vi "runBraking.vi"(6 "Fault?":bool, 7 "x acceleration":dbl, 8 "error in (no error)":errorcluster, 9 "Actuators in":T1, 10 "State in":T2, 11 "SystemsCheck in":refnum<class "SystemsCheck.lvclass">) -> (0 "error out":errorcluster, 1 "Actuators out":T1, 2 "State out":T2, 3 "SystemsCheck out":refnum<class "SystemsCheck.lvclass">)   [LabVIEW 2017, in "ControlLibrary.lvlib" / "SystemsCheck.lvclass"]
uses:
  SystemsCheck.lvclass
  TypeDef_ControlState.ctl
  TypeDef_DigitalOuts.ctl
  RunTypeClass/RunType.lvclass
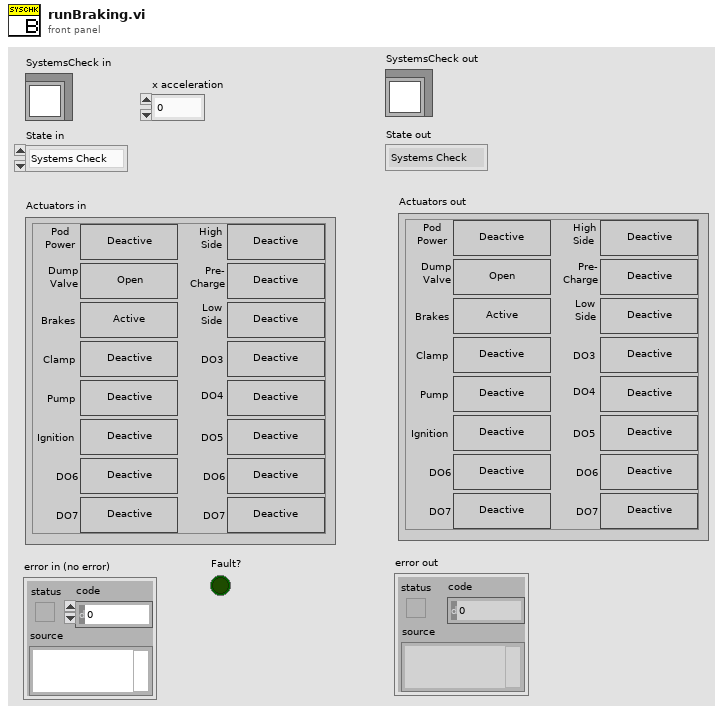
[diagram p1: front panel]
types:
  T1 = typedef "TypeDef_DigitalOuts.ctl" = cluster{"Pod Power":bool, "Dump Valve":bool, "Brakes":bool, "Clamp":bool, "Pump":bool, "Ignition":bool, "DO6":bool, "DO7":bool, "HighSide":bool, "Precharge":bool, "LowSide":bool, "DO3":bool, "DO4":bool, "DO5":bool, "DO62":bool, "DO72":bool}
  T2 = typedef "TypeDef_ControlState.ctl" = enum16{"Systems Check", "Idle", "Ready", "Pushing", "Coast", "Braking", "Fault", "Shutdown", "Service", "Precharge", "Blank"}
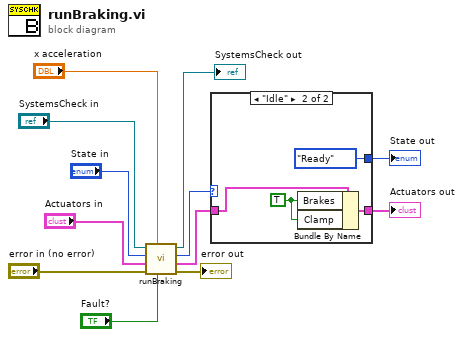
[diagram p0: block diagram]
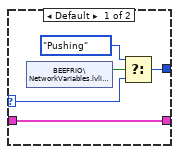
[diagram p2: hidden frame]
diagram:
  n1 = call-parent "runBraking.vi"("Fault?"="Fault?", "x acceleration"="x acceleration", "error in (no error)"="error in (no error)", "Actuators in"="Actuators in", "State in"="State in", "RunType in"="SystemsCheck in") -> ("error out"=→"error out":errorcluster, "Actuators out"=w3:T1, "State out"=w4:T2, "RunType out"=→"SystemsCheck out":refnum<class "SystemsCheck.lvclass">)  [unwired: 2 in]
  n2 = case shown="\"Idle\"" w4 {
    selector: w4 -> [w16 _]
    tunnel: w3 -> [w17 w19]
    tunnel: [w17 w20] -> w2
    tunnel: [w15 TypeDef_ControlState."Ready" ("State out")] -> w1
    frame Default {
      n3 = shared-variable "BEEFRIO\\NetworkVariables.lvlib\\Service"() -> (w14:bool)  [unwired: 1 in, 1 out]
      n4 = Select(t=TypeDef_ControlState."Pushing", s=w14, f=w16) -> (s? t:f=w15:T2)
    }
    frame "Idle" {
      w18 = TRUE ("Actuators.Brakes")
      n5 = Bundle By Name(cluster=w19, "Brakes"=w18, "Clamp"=w18) -> (w20:T1)
    }
  }
  "Actuators out" <- w2
  "State out" <- w1
